vi "Splash Screen.vi"   [LabVIEW 2016]
types:
  T1 = enum32{"Invalid", "Standard", "Closed", "Hidden", "Minimized", "Maximized"}
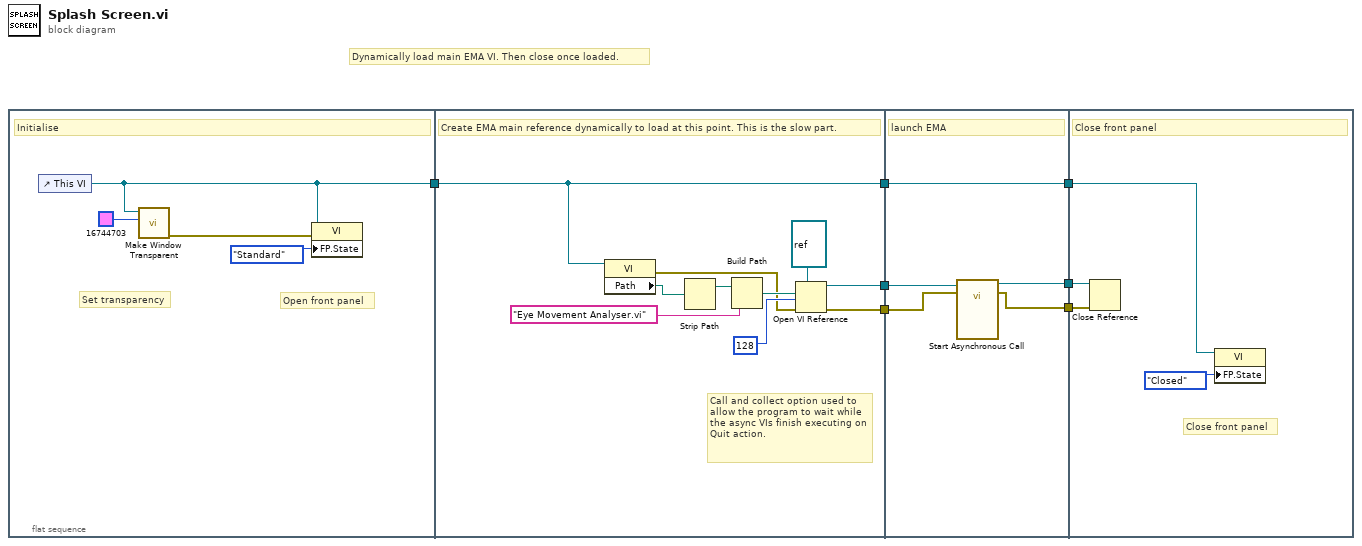
[diagram p0: block diagram]
diagram:
  # "Dynamically load main EMA VI. Then close once loaded."
  n1 = flat-sequence {
    tunnel: [w8] -> w6
    tunnel: [w19] -> w7
    tunnel: w6 -> [w13]
    tunnel: [w13] -> w4
    tunnel: [w12] -> w2
    tunnel: w7 -> [w26]
    tunnel: [w25] -> w5
    tunnel: w4 -> [w24]
    tunnel: [w24] -> w3
    tunnel: w2 -> [w23]
    tunnel: [w22] -> w1
    tunnel: w5 -> [w28]
    tunnel: w3 -> [w29]
    tunnel: w1 -> [w27]
    frame #0 {
      # "Open front panel"
      # "Set transparency"
      # "Initialise"
      n2 = control-ref of="This VI"() -> (w8:refnum<vi>)
      n3 = call <vilib>:"Make Window Transparent.vi"("Colour"=u32 16744703, "VI Refnum"=w8) -> ("error out"=w9:errorcluster)  [unwired: 9 in]
      n4 = property class="VI"(reference=w8, error in=w9, "FP.State"=T1."Standard" ("Front Panel Window:State")) -> ()  [unwired: 2 out]
    }
    frame #1 {
      # "Call and collect option used to allow the program to wait while the async VIs finish executing on Quit action."
      # "Create EMA main reference dynamically to load at this point. This is the slow part."
      n5 = property class="VI"(reference=w13) -> (error out=w17:errorcluster, "Path"=w15:path)  [unwired: 1 in, 1 out]
      n6 = Strip Path(path=w15) -> (stripped path=w14:path)  [unwired: 1 out]
      n7 = Build Path(base path=w14, name or relative path="Eye Movement Analyser.vi") -> (appended path=w18:path)
      n8 = Open VI Reference(type specifier VI Refnum (for type only)=refnum<vi> refnum, vi path=w18, options=128, error in (no error)=w17) -> (vi reference=w19:refnum<vi>, error out=w12:errorcluster)  [unwired: 2 in]
    }
    frame #2 {
      # "launch EMA"
      n9 = call-by-ref "Start Asynchronous Call"(reference=w26, error in=w23) -> (reference out=w25:refnum<vi>, error out=w22:errorcluster)  [unwired: 8 in]
    }
    frame #3 {
      # "Close front panel"
      # "Close front panel"
      n10 = Close Reference(reference=w28, error in (no error)=w27) -> ()  [unwired: 1 out]
      n11 = property class="VI"(reference=w29, "FP.State"=T1."Closed" ("Front Panel Window:State")) -> ()  [unwired: 1 in, 2 out]
    }
  }
